vi "Configuration - Load Module Settings.vi"(7 "section":string, 8 "error in":errorcluster, 10 "Device Type":T2, 11 "Refnum in":T3) -> (0 "error out":errorcluster, 2 "Module Configuration":T1, 3 "Refnum out":T3)   [LabVIEW 2017, in "Communications Library.lvlib"]
uses:
  Communications Library.lvlib
  <vilib>/Utility/config.llb/Config Data RefNum.ctl
  Typedefs/DTACQ Device Type--Enum.ctl
  Typedefs/DTACQ Module Configuration--Cluster.ctl
  <vilib>/Utility/config.llb/Read Key (String).vi
  <vilib>/Utility/config.llb/Read Key (I32).vi
  <vilib>/Utility/config.llb/NI_LVConfig.lvlib
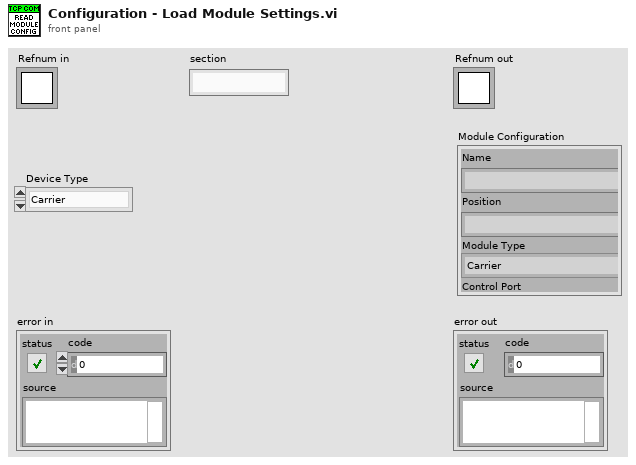
[diagram p1: front panel]
types:
  T1 = typedef "Communications Library.lvlib/DTACQ Module Configuration--Cluster.ctl" = cluster{"Name":string, "Position":string, "Module Type":T2, "Control Port":i32, "Timeout (ms)":i32, "Channels":i32}
  T2 = typedef "Communications Library.lvlib/DTACQ Device Type--Enum.ctl" = enum16{"Carrier", "Analog In Module", "Analog Out Module", "Generic Module"}
  T3 = typedef "NI_LVConfig.lvlib/Config Data RefNum.ctl" = refnum<k1>
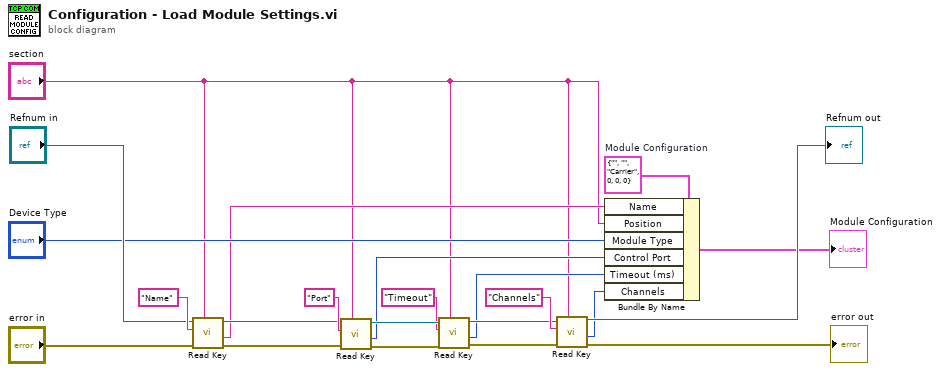
[diagram p0: block diagram]
diagram:
  w8 = T1 {"Name"="", "Position"="", "Module Type"=enum."Carrier", "Control Port"=0, "Timeout (ms)"=0, "Channels"=0}  # Module Configuration
  n1 = call-poly <vilib>:"Read Key.vi"("section"="section", "error in (no error)"="error in", "key"="Name", "refnum"="Refnum in") -> ("error out"=w13:errorcluster, "value"=w6:string, "refnum out"=w14:T3)  [unwired: 4 in, 1 out]
  n2 = call-poly <vilib>:"Read Key.vi"("section"="section", "error in (no error)"=w13, "key"="Port", "refnum"=w14) -> ("error out"=w18:errorcluster, "value"=w5:i32, "refnum out"=w19:T3)  [unwired: 4 in, 1 out]
  n3 = call-poly <vilib>:"Read Key.vi"("section"="section", "error in (no error)"=w18, "key"="Timeout", "refnum"=w19) -> ("error out"=w9:errorcluster, "value"=w4:i32, "refnum out"=w10:T3)  [unwired: 4 in, 1 out]
  n4 = call-poly <vilib>:"Read Key.vi"("section"="section", "error in (no error)"=w9, "key"="Channels", "refnum"=w10) -> ("error out"=→"error out":errorcluster, "value"=w3:i32, "refnum out"=→"Refnum out":T3)  [unwired: 4 in, 1 out]
  n5 = Bundle By Name(cluster=w8, "Name"=w6, "Position"="section", "Module Type"="Device Type", "Control Port"=w5, "Timeout (ms)"=w4, "Channels"=w3) -> (→"Module Configuration":T1)
